vi "Arterial pressure to HR.vi"(10 "Numeric":dbl, 11 "Raw HR":dbl[](array[numeric])) -> (3 "HR":dbl[](array[numeric]))   [LabVIEW 2014]
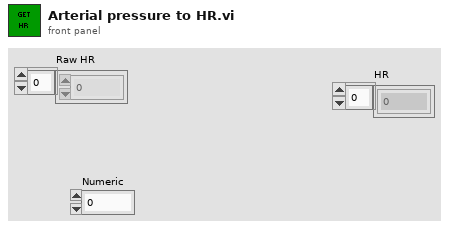
[diagram p1: front panel]
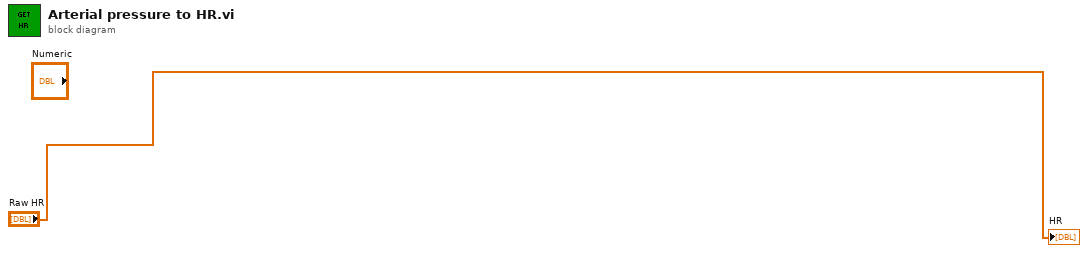
[diagram p0: block diagram]
diagram:
  "HR" <- "Raw HR"
